vi "get_DAQmx_devices_info.vi"(8 "error in":errorcluster) -> (0 "error out":errorcluster, 2 "device count":i32, 3 "Table":string[][](table))   [LabVIEW 2010]
doc: "This VI queries the system information for the device names, product info, and serial number of any National Instruments product installed on your system.\n\nThis VI uses the NI-DAQmx driver software."
uses:
  Program Files/National Instruments/LabVIEW 2010/resource/objmgr/daqmx.rc
panel:
  # "This VI queries the system information for the device names, product info, and serial \nnumber of any National Instruments product installed on your system.\n\nThis VI uses the NI-DAQmx driver software."
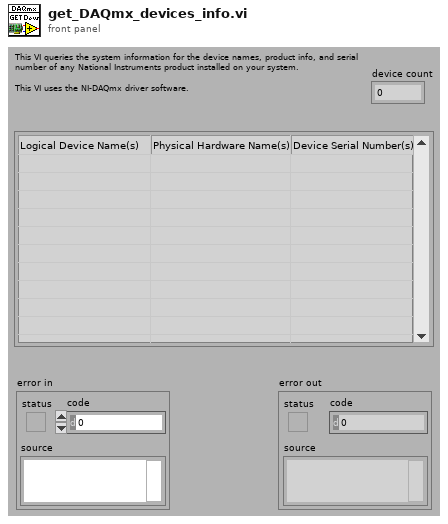
[diagram p1: front panel]
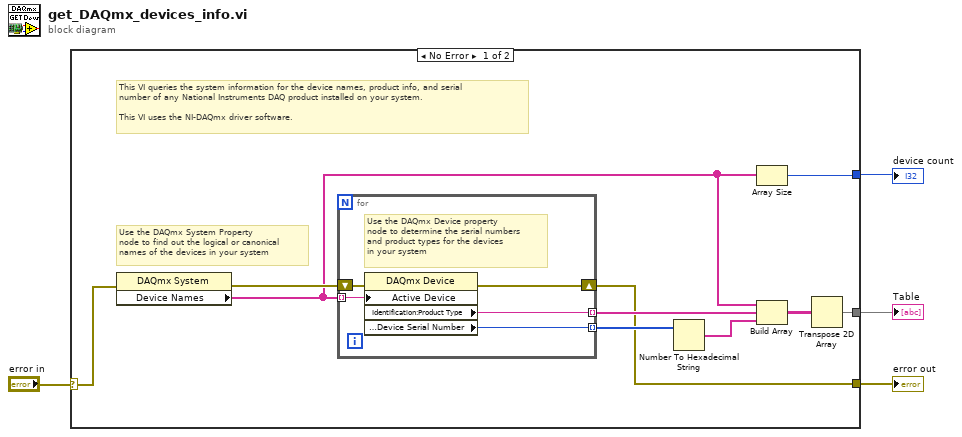
[diagram p0: block diagram]
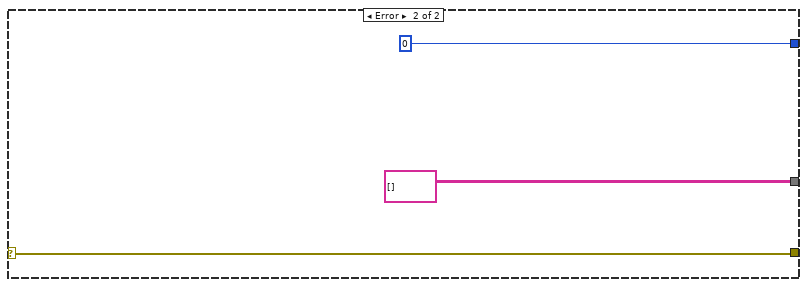
[diagram p2: hidden frame]
diagram:
  n1 = case shown="No Error" "error in" {
    selector: "error in" -> [w5 w22]
    tunnel: [w10 string[][] []] -> w4
    tunnel: [w7 0] -> w3
    tunnel: [w6 w22] -> w2
    frame No Error {
      # "This VI queries the system information for the device names, product info, and serial \nnumber of any National Instruments DAQ product installed on your system.\n\nThis VI uses the NI-DAQmx driver software."
      # "Use the DAQmx System Property\nnode to find out the logical or canonical\nnames of the devices in your system"
      n2 = property class="DAQmx System"(error in=w5) -> (error out=w9:errorcluster, "Device Names"=w8:tag[])  [unwired: 1 in, 1 out]
      n3 = for {
        tunnel: w8 -> [w19] mode=indexing
        tunnel: [w18] -> w12 mode=indexing
        tunnel: [w17] -> w14 mode=indexing
        shift-right: [w15] -> w6
        shift-left: w9 -> [w16]
        # "Use the DAQmx Device property\nnode to determine the serial numbers\nand product types for the devices\nin your system"
        n4 = property class="DAQmx Device"(error in=w16, "Active Device"=w19) -> (error out=w15:errorcluster, "Identification:Product Type"=w18:string, "Identification:Device Serial Number"=w17:u32)  [unwired: 1 in, 1 out]
      }
      n5 = Number To Hexadecimal String(2:w14) -> (0:w13:string[])  [unwired: 1 in]
      n6 = Array Size(array=w8) -> (size(s)=w7:i32)
      n7 = Build Array(w8, w12, w13) -> (w11:string[][])
      n8 = Transpose 2D Array(2D array=w11) -> (transposed array=w10:string[][])
    }
    frame Error {
    }
  }
  "Table" <- w4
  "device count" <- w3
  "error out" <- w2
